vi "initialize.vi"(6 "TaskRef in":refnum<vi>, 8 "error in":errorcluster, 11 "pdbm_task_data":T3) -> (0 "error out":errorcluster, 2 "pdbm_task_data":T2, 3 "pdbm_task_event":T1, 4 "TaskRef out":refnum<vi>, 5 "pdbm_task_reg_reqst_event":refnum<event-registration>)   [LabVIEW 2015, in "pdbm_tasks.lvlib"]
uses:
  pdbm_tasks.lvlib
  pdbm_test_route/UsrDefine/TaskFeedbackCmd.ctl
  pdbm_test_route/UsrDefine/TaskReqst.ctl
  UsrDefine/PDBM_TestSystem_Data.ctl
  pdbm_test_route/pdbm_task_route.lvlib
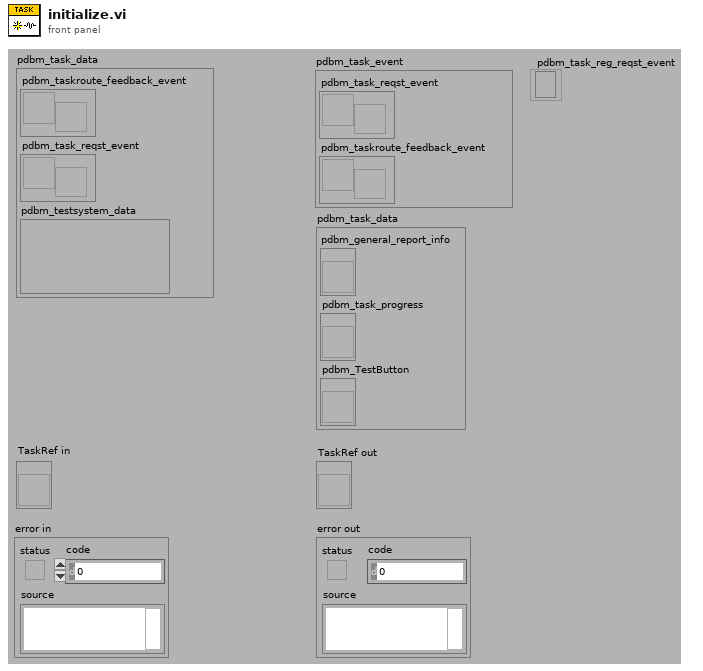
[diagram p1: front panel]
types:
  T1 = cluster{"pdbm_task_reqst_event":refnum<user-event>, "pdbm_taskroute_feedback_event":refnum<user-event>}
  T2 = typedef "pdbm_tasks.lvlib/PDBM_TestSystem_Data.ctl" = cluster{"pdbm_general_report_info":refnum<vi>, "pdbm_task_progress":refnum<vi>, "pdbm_TestButton":refnum<vi>}
  T3 = cluster{"pdbm_taskroute_feedback_event":refnum<user-event>, "pdbm_task_reqst_event":refnum<user-event>, "pdbm_testsystem_data":variant}
  T4 = cluster{"pdbm_task_reqst_event":refnum<user-event>, "pdbm_taskroute_feedback_event out":refnum<user-event>}
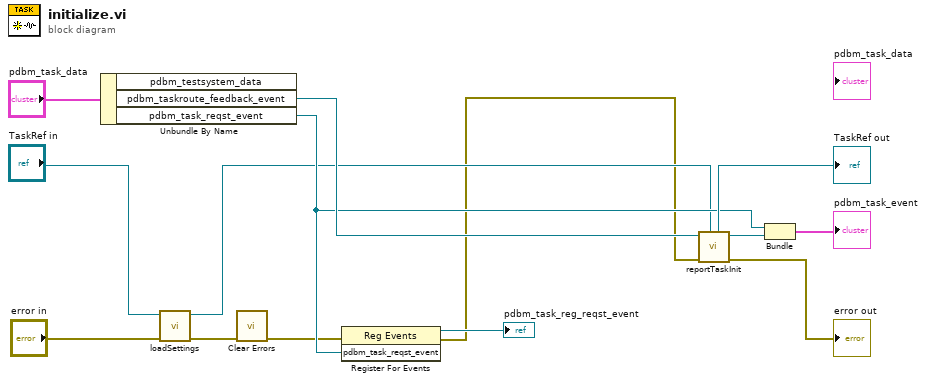
[diagram p0: block diagram]
diagram:
  n1 = Unbundle By Name("pdbm_task_data") -> ("pdbm_taskroute_feedback_event"=w13:refnum<user-event>, "pdbm_task_reqst_event"=w10:refnum<user-event>)  [unwired: 1 out]
  n2 = call "loadSettings.vi"("error in (no error)"="error in", "TaskRef in"="TaskRef in") -> ("error out"=w5:errorcluster, "TaskRef out"=w3:refnum<vi>)  [unwired: 8 in]
  n3 = call <vilib>:"Clear Errors.vi"("error in (no error)"=w5) -> ("error out"=w2:errorcluster)  [unwired: 5 in, 1 out]
  n4 = register-events(error in=w2, w10) -> (reference out=→"pdbm_task_reg_reqst_event":refnum<event-registration>, error out=w1:errorcluster)  [unwired: 1 in]
  n5 = call "reportTaskInit.vi"("TaskRef"=w3, "error in (no error)"=w1, "pdbm_taskroute_feedback_event"=w13) -> ("error out"=→"error out":errorcluster, "pdbm_taskroute_feedback_event out"=w11:refnum<user-event>, "TaskRef out"=→"TaskRef out":refnum<vi>)  [unwired: 6 in]
  n6 = Bundle("pdbm_task_reqst_event"=w10, "pdbm_taskroute_feedback_event out"=w11) -> (→"pdbm_task_event":T4)  [unwired: 1 in]
